vi "Compute_the_given_expression.vi"() -> ()   [LabVIEW 2020]
panel:
  in  "c":dbl
  in  "x":dbl
  in  "m":dbl
  in  "E":dbl
  in  "D":dbl
  in  "C":dbl
  in  "B":dbl
  in  "A":dbl
  out "Y = mx+c":dbl
  out "Y=(A*B*C)+(D*E)":dbl
  # "Compute the expressions Y=(A*B*C)+(D*E) and Y=mx+c"
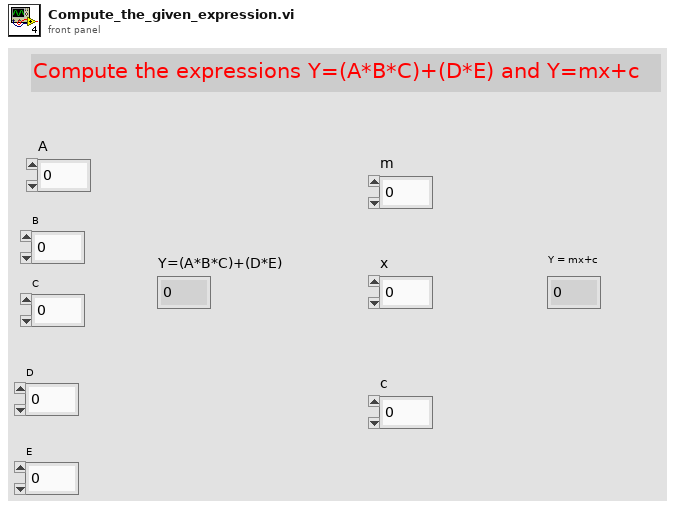
[diagram p1: front panel]
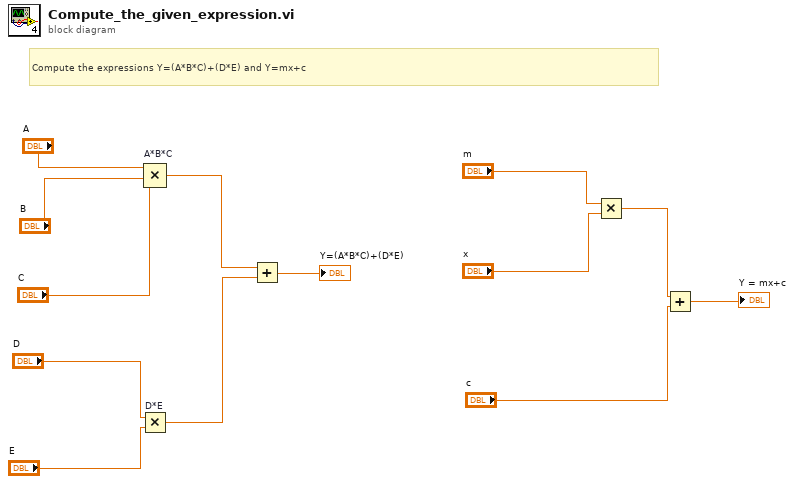
[diagram p0: block diagram]
diagram:
  # "Compute the expressions Y=(A*B*C)+(D*E) and Y=mx+c"
  n1 = Multiply "D*E"(x="D", y="E") -> (x*y=w7:dbl)
  n2 = Compound Arithmetic op=MULTIPLY "A*B*C"("A", "B", "C") -> (w8:dbl)
  n3 = Add(x=w8, y=w7) -> (x+y=→"Y=(A*B*C)+(D*E)":dbl)
  n4 = Multiply(x="m", y="x") -> (x*y=w2:dbl)
  n5 = Add(x=w2, y="c") -> (x+y=→"Y = mx+c":dbl)
